vi "BoilerPlate.vi"(5 "Teleop Local Data In":T1, 9 "error in":errorcluster) -> (6 "Teleop Local Data Out":T1, 10 "error out":errorcluster)   [LabVIEW 2019]
uses:
  Typedefs/typedef_cluster_TeleOp_Local_Data.ctl
  Typedefs/typedef_cluster_Joystick.ctl
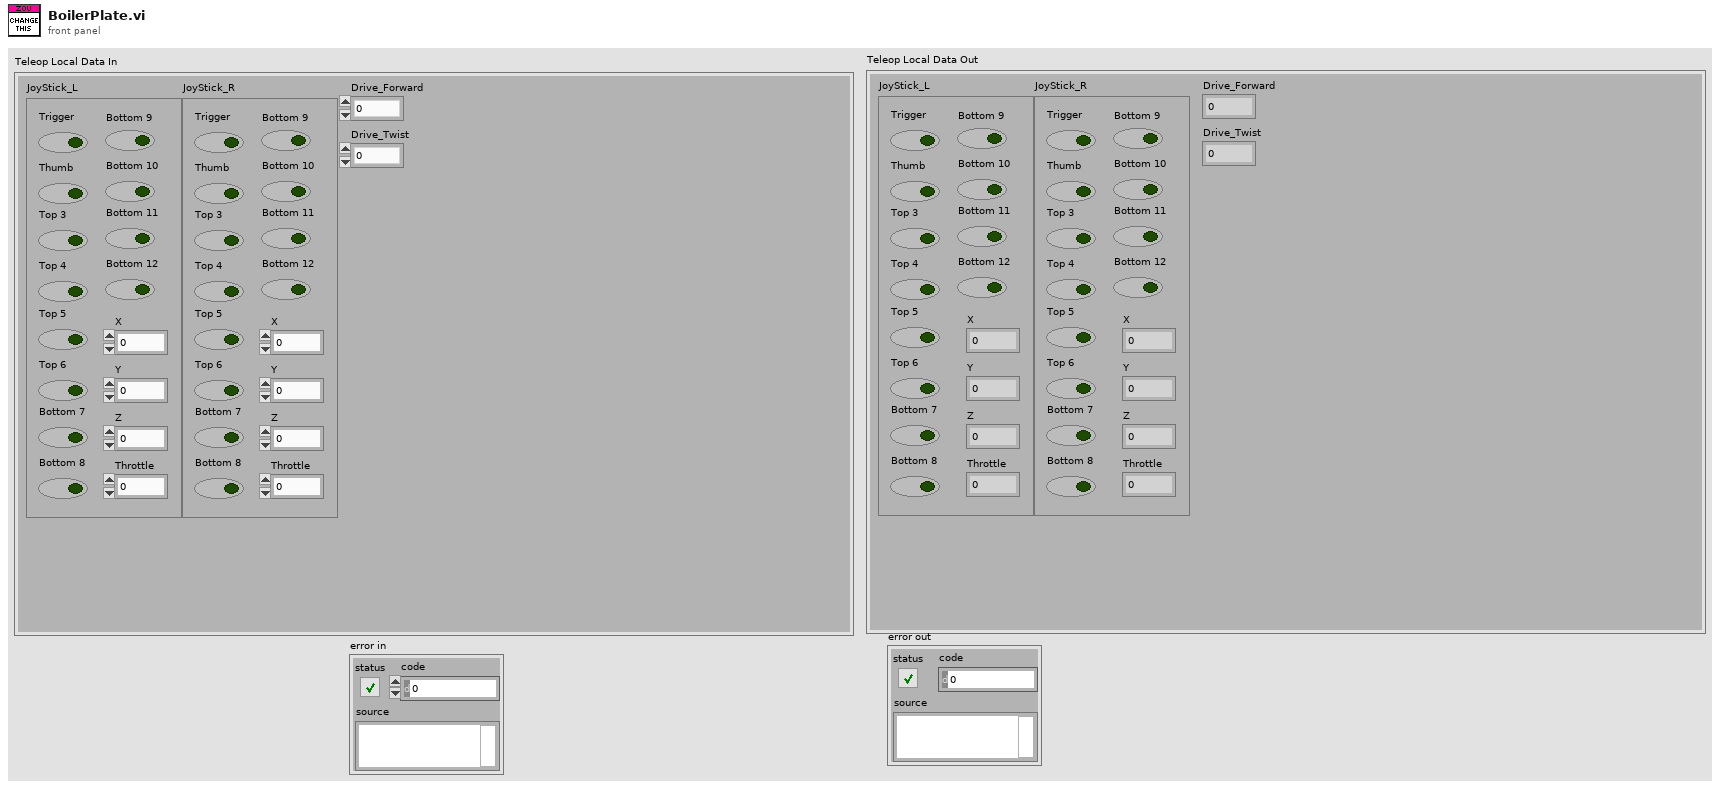
[diagram p1: front panel]
types:
  T1 = typedef "typedef_cluster_TeleOp_Local_Data.ctl" = cluster{"JoyStick_L":T2, "JoyStick_R":T2, "Drive_Forward":dbl, "Drive_Twist":dbl}
  T2 = typedef "typedef_cluster_Joystick.ctl" = cluster{"X":dbl, "Y":dbl, "Z":dbl, "Throttle":dbl, "Trigger":bool, "Thumb":bool, "Top 3":bool, "Top 4":bool, "Top 5":bool, "Top 6":bool, "Bottom 7":bool, "Bottom 8":bool, "Bottom 9":bool, "Bottom 10":bool, "Bottom 11":bool, "Bottom 12":bool}
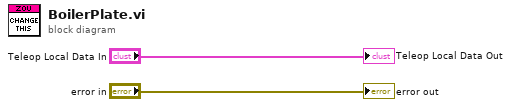
[diagram p0: block diagram]
diagram:
  "Teleop Local Data Out" <- "Teleop Local Data In"
  "error out" <- "error in"
